vi "viewer.vi"() -> ()   [LabVIEW 2017]
uses:
  <vilib>/Utility/file.llb/Read Delimited Spreadsheet (DBL).vi
panel:
  out "Numeric 2":dbl
  in  "Numeric":dbl
  out "Waveform Graph":dbl[](graph)
  in  "file path (dialog if empty)":path
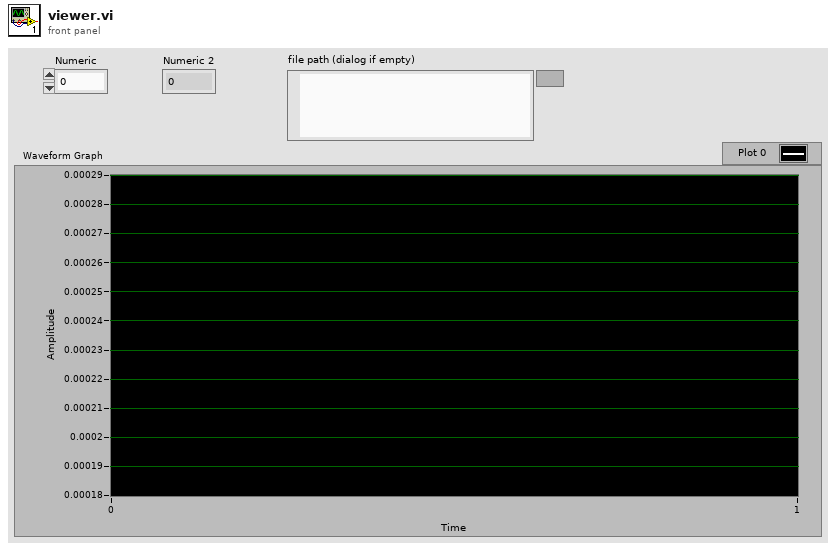
[diagram p1: front panel]
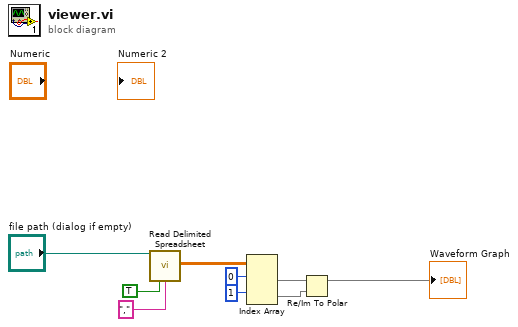
[diagram p0: block diagram]
diagram:
  n1 = call-poly <vilib>:"Read Delimited Spreadsheet.vi"("file path (dialog if empty)"="file path (dialog if empty)", "transpose? (F)"=TRUE, "delimiter (\\t)"="," ("delimiter (\\t)")) -> ("all rows"=w7:dbl[][])  [unwired: 7 in, 5 out]
  n2 = Index Array(array=w7, index (row) #1=0 ("index (row)"), index (row) #2=1 ("index (row)")) -> (element #1=w5:dbl[], element #2=w3:dbl[])  [unwired: 2 in]
  n3 = Re/Im To Polar(2:w3, 3:w5) -> (1:→"Waveform Graph":dbl[])  [unwired: 1 out]
